vi "Write Port Out L.vi"(8 "error in (no error)":errorcluster caption="错误输入（无错误）", 10 "out_port":u8, 11 "dev":i32) -> (0 "error out":errorcluster caption="错误输出", 3 "function return":i32)   [LabVIEW 2018, in "恒凯采集卡.lvlib"]
doc: "int Write_Port_OutL(int dev,unsigned char out_port);"
uses:
  data/Usb_Daq_V52_32.dll
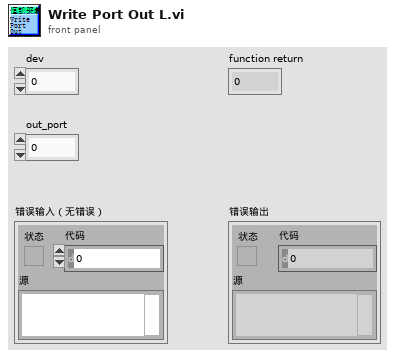
[diagram p1: front panel]
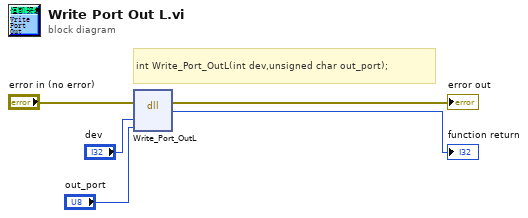
[diagram p0: block diagram]
diagram:
  # "int Write_Port_OutL(int dev,unsigned char out_port);"
  n1 = dll-call lib="D:/ProgramFiles/NI/LabVIEW 2018/user.lib/Usb_Daq_V52_32/Usb_Daq_V52_32.*" fn="Write_Port_OutL"(error in="error in (no error)", "dev"="dev", "out_port"="out_port") -> (error out=→"error out":errorcluster, →"function return":i32)  [unwired: 4 in, 1 out]
